vi "MGCC_EnergyMgmt_GC_objconstraint_fcns.vi"(9 "output selector":T1, 10 "data":variant, 11 "X":dbl[](array[numeric])) -> (0 "error out":errorcluster, 1 "inequality constraint function values":dbl[](array[numeric]), 2 "equality constraint function values":dbl[](array[numeric]), 3 "objective function value":dbl)   [LabVIEW 2016]
doc: "This template is the starting point for creating an objective function, equality constraint function and inequality constraint function to be passed to the Constrained Nonlinear Optimization.vi."
uses:
  <vilib>/gmath/NumericalOptimization/cno_output select.ctl
  <vilib>/imath/engines/lvmath2/RunTimeEngine/ArithmeticOperatorToken/NIMS_ArithmeticOperator_minus.vi
  <instcachedir>/0/NIMS_ArithmeticOperator_minus_E3B65B1D26A44BB184AFDC5B3F458E3D.lvgen/NIMS_ArithmeticOperator_minus_E3B65B1D26A44BB184AFDC5B3F458E3D_002.vi
  <vilib>/imath/engines/lvmath2/RunTimeEngine/BuiltInFunctions/max/1 input/NIMS_max(RM).vi
  <instcachedir>/0/NIMS_max(RM)_358AE92FF7FA4D91BF0D9DEC69043403.lvgen/NIMS_max(RM)_358AE92FF7FA4D91BF0D9DEC69043403_000.vi
  <vilib>/imath/engines/lvmath2/RunTimeEngine/ArithmeticOperatorToken/NIMS_ArithmeticOperator_multmx.vi
  <instcachedir>/0/NIMS_ArithmeticOperator_multmx_4A56FE5C615140CE835D4DB5891BF065.lvgen/NIMS_ArithmeticOperator_multmx_4A56FE5C615140CE835D4DB5891BF065_004.vi
  <vilib>/imath/engines/lvmath2/RunTimeEngine/ArithmeticOperatorToken/NIMS_ArithmeticOperator_plus.vi
  <instcachedir>/0/NIMS_ArithmeticOperator_plus_0120E0498A0F4B4B9BDCAC2554767A4E.lvgen/NIMS_ArithmeticOperator_plus_0120E0498A0F4B4B9BDCAC2554767A4E_003.vi
  <vilib>/imath/engines/lvmath2/RunTimeEngine/BuiltInFunctions/max/1 input/NIMS_max(RV).vi
  <instcachedir>/0/NIMS_max(RV)_237633DB1D604D5BA7001287DF3C7957.lvgen/NIMS_max(RV)_237633DB1D604D5BA7001287DF3C7957_000.vi
  <vilib>/imath/engines/lvmath2/RunTimeEngine/ErrorHandling/NIMS_Create Error From Enums.vi
  <vilib>/imath/engines/lvmath2/RunTimeEngine/ArithmeticOperatorToken/NIMS_ArithmeticOperator_multmx(M,CV).vi
  <instcachedir>/0/NIMS_ArithmeticOperator_multmx(M,CV)_EE734FC8520844C9A7CC1A67008668A3.lvgen/NIMS_ArithmeticOperator_multmx(M,CV)_EE734FC8520844C9A7CC1A67008668A3_000.vi
  <vilib>/imath/engines/lvmath2/RunTimeEngine/IndexRead/NIMS M($,S).vi
  <instcachedir>/0/NIMS M($,S)_3E5749BBB62E49528D4765A77F1F6D98.lvgen/NIMS M($,S)_3E5749BBB62E49528D4765A77F1F6D98_000.vi
  <vilib>/imathl/engines/lvmath/Functions/Error Handling/Create Error.vi
  <vilib>/imath/engines/lvmath2/RunTimeEngine/NodeEndStatement/NIMS_NodeEndStatement_Output.vi
  <instcachedir>/0/NIMS_NodeEndStatement_Output_53EC0D466D134D7ABD903AC30B43404B.lvgen/NIMS_NodeEndStatement_Output_53EC0D466D134D7ABD903AC30B43404B_005.vi
  <instcachedir>/0/NIMS_NodeEndStatement_Output_53EC0D466D134D7ABD903AC30B43404B.lvgen/NIMS_NodeEndStatement_Output_53EC0D466D134D7ABD903AC30B43404B_001.vi
  <vilib>/imath/engines/lvmath2/RunTimeEngine/ErrorHandling/NIMS_Finalize Error.vi
  <vilib>/gmath/NI_Gmath.lvlib
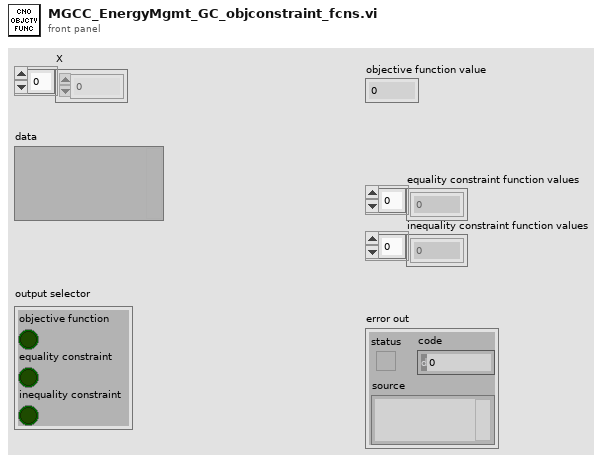
[diagram p1: front panel]
types:
  T1 = typedef "NI_Gmath.lvlib/cno_output select.ctl" = cluster{"objective function":bool, "equality constraint":bool, "inequality constraint":bool}
  T2 = cluster{"Load24":dbl[], "PV24":dbl[], "Price":dbl[], "DemandPrice":dbl, "A":dbl[][], "E0":dbl}
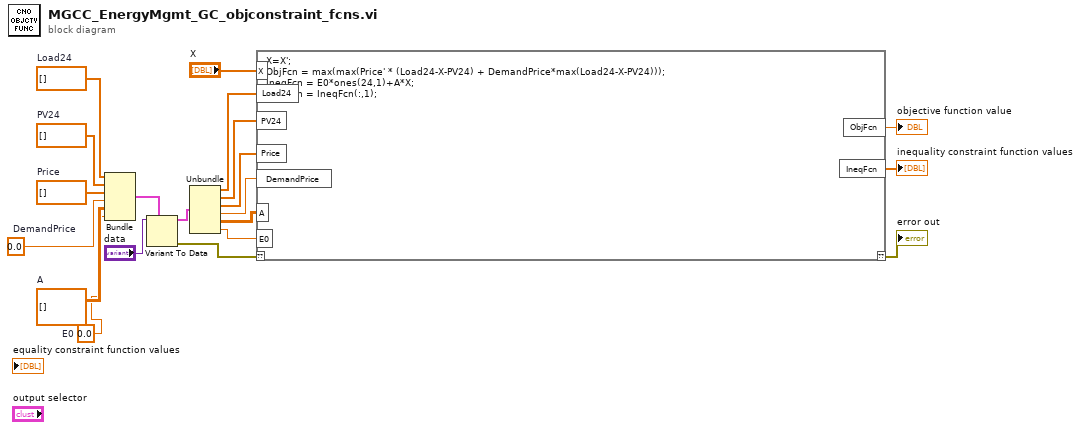
[diagram p0: block diagram]
diagram:
  w2 = 0.0  # E0
  w18 = 0.0  # DemandPrice
  w19 = dbl[] []  # Price
  w20 = dbl[] []  # PV24
  w13 = dbl[] []  # Load24
  w17 = dbl[][] []  # A
  n1 = Bundle("Load24"=w13, "PV24"=w20, "Price"=w19, "DemandPrice"=w18, "A"=w17, "E0"=w2) -> (w15:T2)  [unwired: 1 in]
  n2 = Variant To Data(type=w15, Variant="data") -> (data=w14:T2, error out=w12:errorcluster)  [unwired: 1 in]
  n3 = Unbundle(w14) -> ("Load24"=w11:dbl[], "PV24"=w10:dbl[], "Price"=w9:dbl[], "DemandPrice"=w8:dbl, "A"=w7:dbl[][], "E0"=w1:dbl)
  n4 = mathscript code="X=X';\nObjFcn = max(max(Price' * (Load24-X-PV24) + DemandPrice*max(Load24-X-PV24))); \nIneqFcn = E0*ones(24,1)+A*X;\nIneqFcn = IneqFcn(:,1);"("??"=w12, "Load24"=w11, "PV24"=w10, "Price"=w9, "DemandPrice"=w8, "A"=w7, "X"="X", "E0"=w1) -> ("??"=→"error out":errorcluster, "ObjFcn"=→"objective function value":dbl, "IneqFcn"=→"inequality constraint function values":dbl[])
